vi "ROSmsg_getParser.vi"(9 "Package Path":path, 10 "Is Array?":bool, 11 "Data Type":string) -> (1 "msg path":path, 3 "Parser Path":path)   [LabVIEW 2015]
doc: "Build the expected path to the parser of this data type."
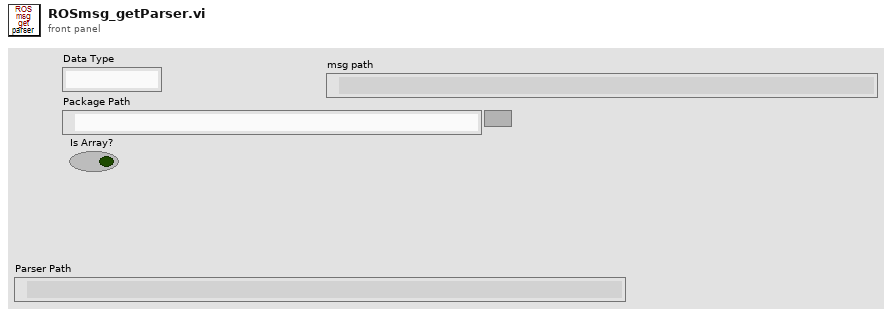
[diagram p1: front panel]
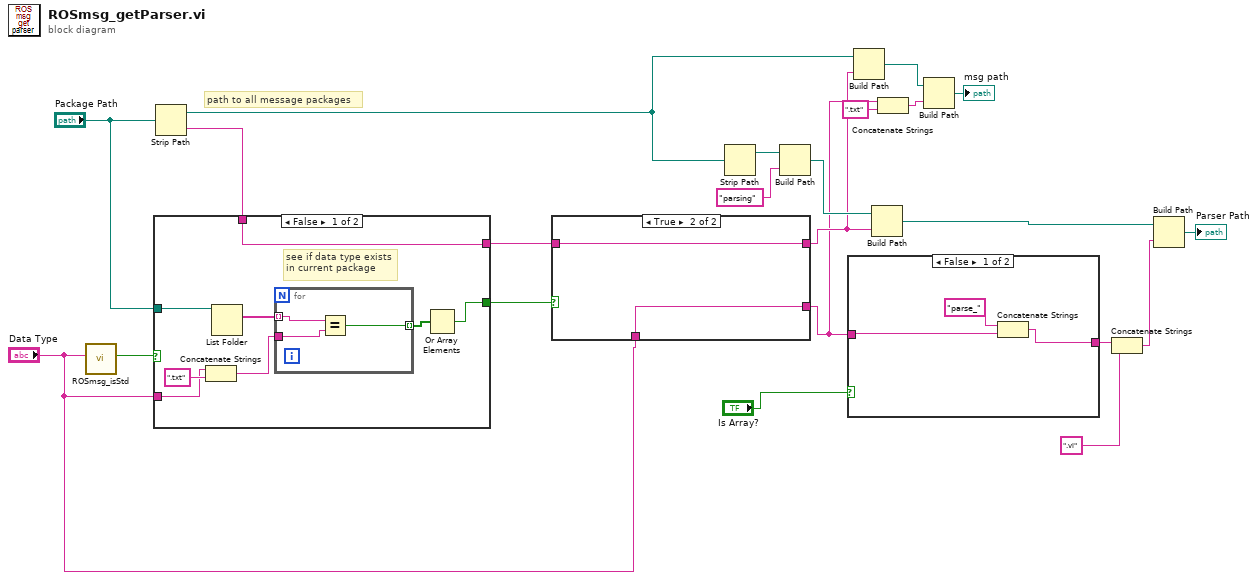
[diagram p0: block diagram]
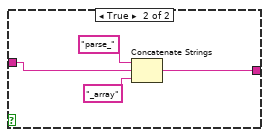
[diagram p2: hidden frame]
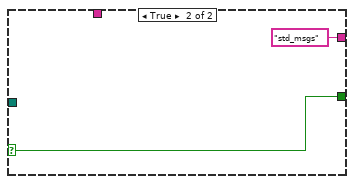
[diagram p3: hidden frame]
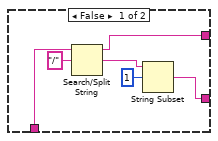
[diagram p4: hidden frame]
diagram:
  # "path to all message packages"
  n1 = call "ROSmsg_isStd.vi"("Data Type"="Data Type") -> ("Is std_msgs?"=w16:bool)  [unwired: 10 in]
  n2 = Strip Path(path="Package Path") -> (stripped path=w7:path, name=w15:string)
  n3 = case shown="False" w16 {
    selector: w16 -> [_ w35]
    tunnel: "Package Path" -> [w30 _]
    tunnel: [w26 w35] -> w17
    tunnel: w15 -> [w25 _]
    tunnel: [w25 "std_msgs" ("name")] -> w14
    tunnel: "Data Type" -> [w24 _]
    frame False {
      # "see if data type exists\nin current package"
      n4 = Concatenate Strings(w24, ".txt" ("string")) -> (w23:string)
      n5 = List Folder(path=w30) -> (filenames=w28:string[])  [unwired: 3 in, 3 out]
      n6 = for {
        tunnel: w28 -> [w33] mode=indexing
        tunnel: w23 -> [w32]
        tunnel: [w31] -> w27 mode=indexing
        n7 = Equal?(x=w33, y=w32) -> (x = y?=w31:bool)
      }
      n8 = Or Array Elements(Boolean array=w27) -> (logical OR=w26:bool)
    }
    frame True {
    }
  }
  n9 = case shown="True" w17 {
    tunnel: w14 -> [_ w43]
    tunnel: [w40 w43] -> w6
    tunnel: "Data Type" -> [w41 w42]
    tunnel: [w37 w42] -> w3
    frame False {
      n10 = Search/Split String(string=w41, search string/char (-)="/") -> (substring before match=w40:string, match + rest of string=w38:string)  [unwired: 1 in, 1 out]
      n11 = String Subset(string=w38, offset (0)=1) -> (substring=w37:string)  [unwired: 1 in]
    }
    frame True {
    }
  }
  n12 = Strip Path(path=w7) -> (stripped path=w20:path)  [unwired: 1 out]
  n13 = Build Path(base path=w20, name or relative path="parsing") -> (appended path=w19:path)
  n14 = case shown="False" "Is Array?" {
    tunnel: w3 -> [w45 w50]
    tunnel: [w44 w47] -> w12
    frame False {
      n15 = Concatenate Strings("parse_" ("string"), w45) -> (w44:string)
    }
    frame True {
      n16 = Concatenate Strings("parse_" ("string"), w50, "_array" ("string")) -> (w47:string)
    }
  }
  n17 = Build Path(base path=w7, name or relative path=w6) -> (appended path=w5:path)
  n18 = Build Path(base path=w19, name or relative path=w6) -> (appended path=w18:path)
  n19 = Concatenate Strings(w3, ".txt" ("string")) -> (w4:string)
  n20 = Build Path(base path=w5, name or relative path=w4) -> (appended path=→"msg path":path)
  n21 = Concatenate Strings(w12, ".vi" ("string")) -> (w10:string)
  n22 = Build Path(base path=w18, name or relative path=w10) -> (appended path=→"Parser Path":path)
